vi "ForceAndReadNew.vi"(0 "object in":refnum<class "MTEC_Async.lvclass">, 2 "Buffer Values":bool=TRUE, 5 "error in (no error)":errorcluster) -> (14 "object out":refnum<class "MTEC_Async.lvclass">, 16 "Cluster":T3 {"DataOut"."meTEC_CH2_Temperature Stability" items=["Temperature regulation is not active", "Is not stable", "Is stable"]; "DataOut"."meTEC_CH1_Device Status" items=["Initializing", "Ready", "Run", "Error", "Bootloader", "Reset in Progress"]; "DataOut"."meTEC_CH1_Temperature Stability" items=["Temperature regulation is not active", "Is not stable", "Is stable"]}, 19 "error out":errorcluster)   [LabVIEW 2019, in "MTEC_Async.lvclass"]
uses:
  MTEC_Async.lvclass
  TEC LabVIEW Control Software v0.14/Source/LV Source/[meerstetter engineering TE Cooling]/TypeDefs/meTEC_ID 1200_Temperature is Stable.ctl
  TEC LabVIEW Control Software v0.14/Source/LV Source/[meerstetter engineering TE Cooling]/TypeDefs/meTEC_ID 104_Device Status.ctl
  MTEC_Async.lvclass/MTEC_Async.ctl
panel:
  out "timed out? 2":bool
  out "timed out?":bool
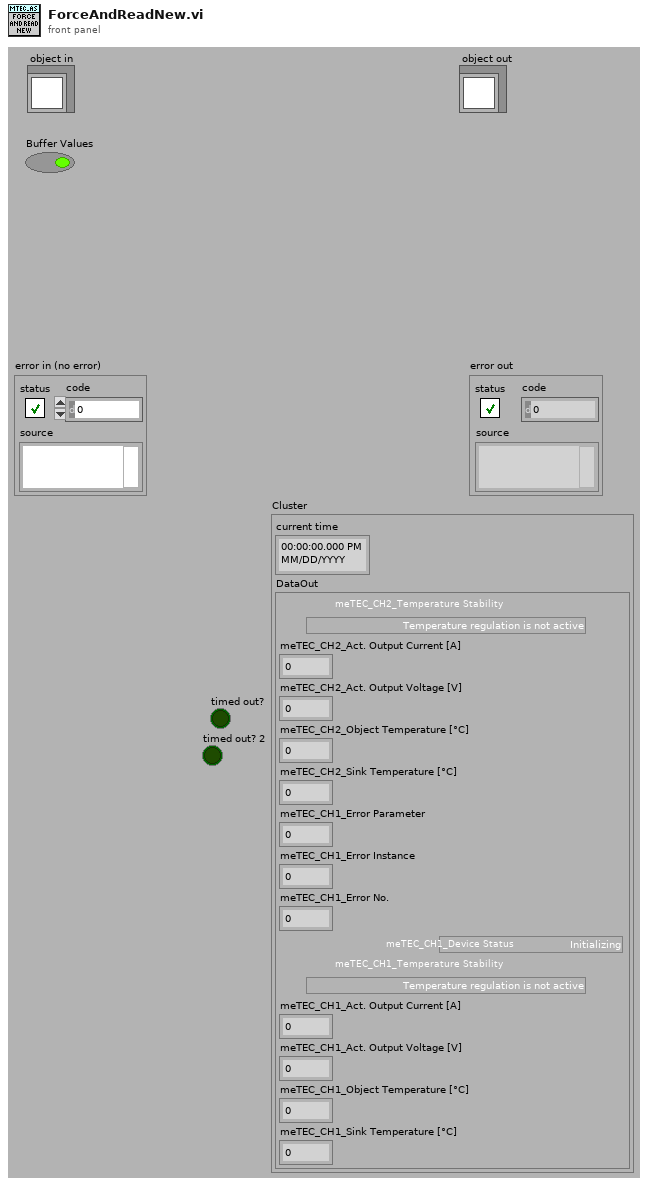
[diagram p1: front panel]
types:
  T1 = typedef "meTEC_ID 1200_Temperature is Stable.ctl" = i32
  T2 = typedef "meTEC_ID 104_Device Status.ctl" = i32
  T3 = cluster{"current time":timestamp, "DataOut":cluster{"meTEC_CH2_Temperature Stability":T1, "meTEC_CH2_Act. Output Current [A]":dbl, "meTEC_CH2_Act. Output Voltage [V]":dbl, "meTEC_CH2_Object Temperature [°C]":dbl, "meTEC_CH2_Sink Temperature [°C]":dbl, "meTEC_CH1_Error Parameter":i32, "meTEC_CH1_Error Instance":i32, "meTEC_CH1_Error No.":i32, "meTEC_CH1_Device Status":T2, "meTEC_CH1_Temperature Stability":T1, "meTEC_CH1_Act. Output Current [A]":dbl, "meTEC_CH1_Act. Output Voltage [V]":dbl, "meTEC_CH1_Object Temperature [°C]":dbl, "meTEC_CH1_Sink Temperature [°C]":dbl}}
  T4 = cluster{"Message":string, "Message Data":variant}
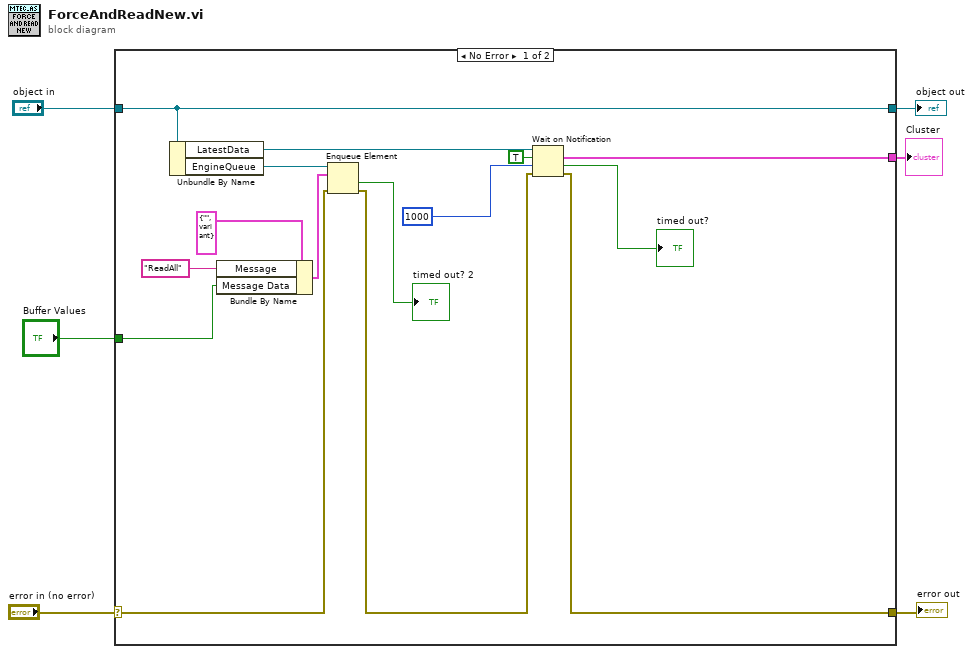
[diagram p0: block diagram]
diagram:
  n1 = case shown="No Error" "error in (no error)" {
    selector: "error in (no error)" -> [w10 w23]
    tunnel: [w16 w23] -> w5
    tunnel: [w21 w22] -> w3
    tunnel: "object in" -> [w21 w22]
    tunnel: [w19 _] -> w1
    tunnel: "Buffer Values" -> [w11 _]
    frame No Error {
      n2 = Unbundle By Name(w21) -> ("LatestData"=w20:refnum<notifier>, "EngineQueue"=w15:refnum<queue>)
      n3 = Bundle By Name(cluster=T4 {"Message"="", "Message Data"=variant} ("element"), "Message"="ReadAll", "Message Data"=w11) -> (w12:T4)
      n4 = Enqueue Element(queue=w15, element=w12, error in (no error)=w10) -> (timed out?=→"timed out? 2":bool, error out=w9:errorcluster)  [unwired: 1 in, 1 out]
      n5 = Wait on Notification(notifier=w20, ignore previous (F)=TRUE, timeout in ms (-1)=1000, error in (no error)=w9) -> (notification=w19:T3, timed out?=→"timed out?":bool, error out=w16:errorcluster)  [unwired: 1 out]
    }
    frame Error {
    }
  }
  "error out" <- w5
  "object out" <- w3
  "Cluster" <- w1
